vi "Tester.vi"() -> ()   [LabVIEW 2020, in "Process Generation.lvlib" / "Process Generator.lvclass"]
uses:
  Process Generator.lvclass
  Framework Test/Process Test/Process Test.lvclass
  Framework/Process/Process.lvclass
  C:/Users/anton/Documents/GitHub/Triarc-Framework/source/Framework Test/Base Class Test/Base Test.lvclass
  C:/Program Files (x86)/National Instruments/LabVIEW 2020/vi.lib/Asteme/LUnit/Test Case.lvclass
  C:/Users/anton/Documents/GitHub/Triarc-Framework/source/Framework Test/Process Test/Process Test.lvclass
panel:
  in  "Numeric":i32
  out "error out":errorcluster
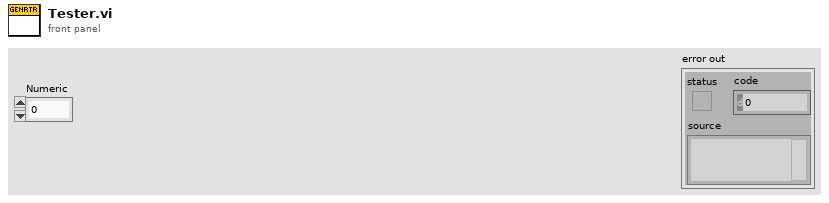
[diagram p1: front panel]
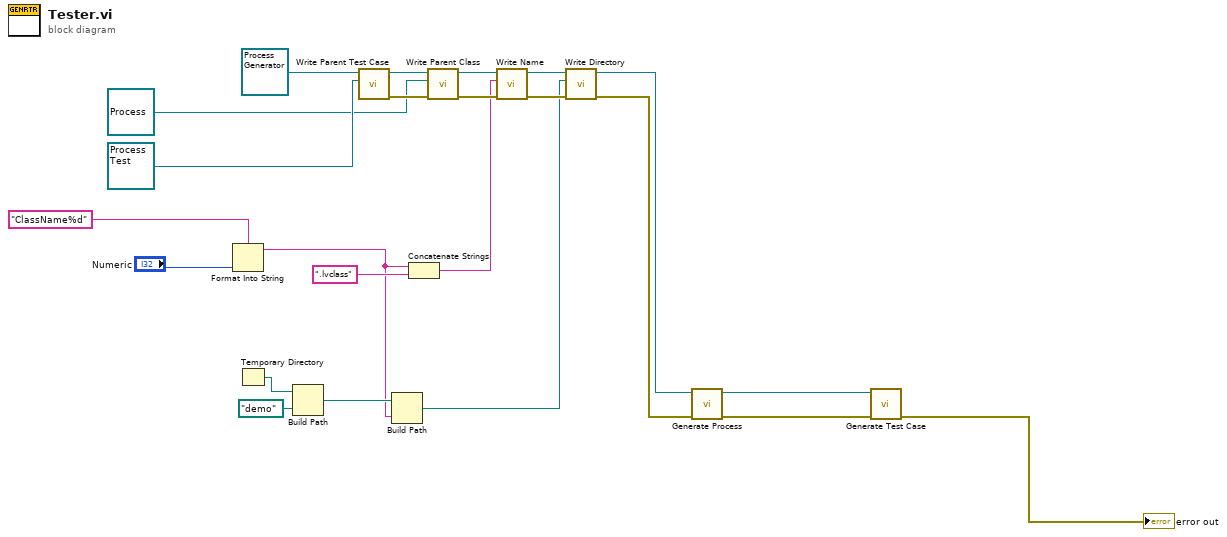
[diagram p0: block diagram]
diagram:
  n1 = Format Into String(format string="ClassName%d", "Numeric") -> (resulting string=w16:string)  [unwired: 2 in, 1 out]
  n2 = Temporary Directory() -> (w23:path)
  n3 = Build Path(base path=w23, name or relative path=path "demo") -> (appended path=w20:path)
  n4 = call "Write Parent Test Case.vi"("Parent Test Case"=refnum<class "Process Test.lvclass"> refnum ("Process Test.lvclass"), "Process Generator In"=refnum<class "Process Generator.lvclass"> refnum) -> ("error out"=w11:errorcluster, "Process Generator Out"=w12:refnum<class "Process Generator.lvclass">)  [unwired: 8 in]
  n5 = Build Path(base path=w20, name or relative path=w16) -> (appended path=w1:path)
  n6 = Concatenate Strings(w16, ".lvclass" ("string")) -> (w2:string)
  n7 = call "Write Parent Class.vi"("error in (no error)"=w11, "Parent Process"=refnum<class "Process.lvclass"> refnum ("Parent Class"), "Process Generator in"=w12) -> ("error out"=w5:errorcluster, "Process Generator out"=w6:refnum<class "Process Generator.lvclass">)  [unwired: 7 in]
  n8 = call "Write Name.vi"("error in (no error)"=w5, "Name"=w2, "Process Generator In"=w6) -> ("error out"=w7:errorcluster, "Process Generator Out"=w8:refnum<class "Process Generator.lvclass">)  [unwired: 7 in]
  n9 = call "Write Directory.vi"("error in (no error)"=w7, "Directory"=w1, "Process Generator in"=w8) -> ("error out"=w3:errorcluster, "Process Generator out"=w4:refnum<class "Process Generator.lvclass">)  [unwired: 7 in]
  n10 = call "Generate Process.vi"("error in (no error)"=w3, "Process Generator In"=w4) -> ("error out"=w18:errorcluster, "Process Generator Out"=w21:refnum<class "Process Generator.lvclass">)  [unwired: 8 in]
  n11 = call "Generate Test Case.vi"("error in (no error)"=w18, "Process Generator In"=w21) -> ("error out"=→"error out":errorcluster)  [unwired: 8 in, 1 out]
